vi "fft aubvi.vi"() -> ()   [LabVIEW 2020]
uses:
  <vilib>/Analysis/2dsp.llb/Real FFT.vi
  <vilib>/Analysis/NI_AALBase.lvlib
  <vilib>/Analysis/NI_AALPro.lvlib
panel:
  out "FFT magnitude":dbl[](graph)
  in  "FFT size":i32=128
  in  "fs [Hz]":dbl
  in  "f0 [Hz]":dbl
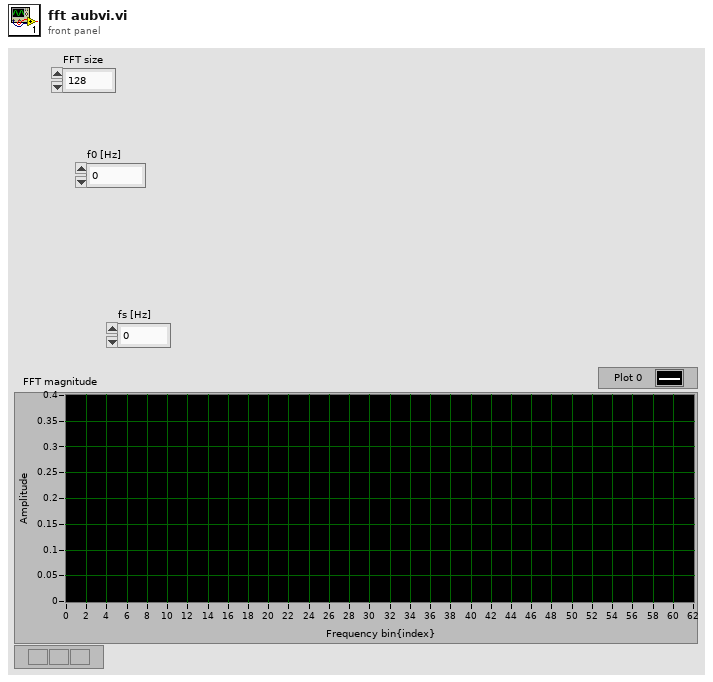
[diagram p1: front panel]
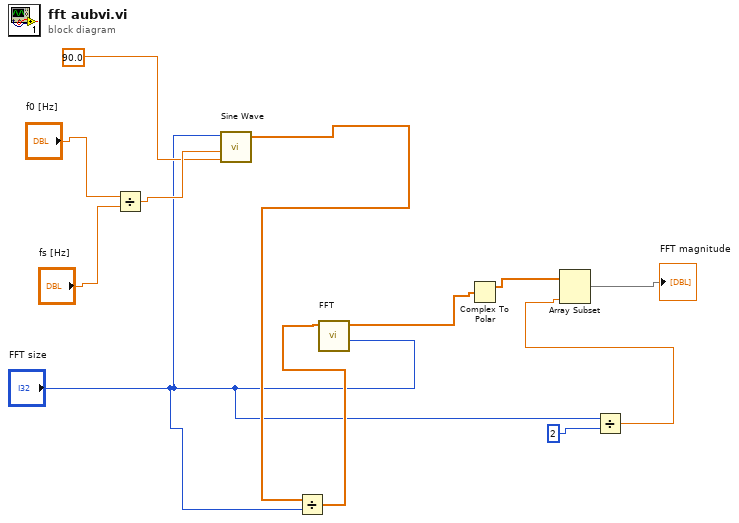
[diagram p0: block diagram]
diagram:
  n1 = Divide(x="f0 [Hz]", y="fs [Hz]") -> (x/y=w12:dbl)
  n2 = call <vilib>:"Sine Wave.vi"("samples"="FFT size", "frequency"=w12, "phase in"=90.0) -> ("sine wave"=w8:dbl[])  [unwired: 2 in, 2 out]
  n3 = Divide(x=w8, y="FFT size") -> (x/y=w7:dbl[])
  n4 = call-poly <vilib>:"FFT.vi"("FFT size"="FFT size", "X"=w7) -> ("FFT {X}"=w6:cdb[])  [unwired: 8 in, 1 out]
  n5 = Complex To Polar(r * e^(i*theta)=w6) -> (r=w5:dbl[])  [unwired: 1 out]
  n6 = Divide(x="FFT size", y=2 ("phase in")) -> (x/y=w1:dbl)
  n7 = Array Subset(array=w5, length=w1) -> (→"FFT magnitude":dbl[])  [unwired: 1 in]
